vi "ConvertToArray.vi"(8 "error in (no error)":errorcluster, 11 "Cluster":T1) -> (0 "error out":errorcluster, 3 "Array":dbl[](array[numeric]))   [LabVIEW 2014]
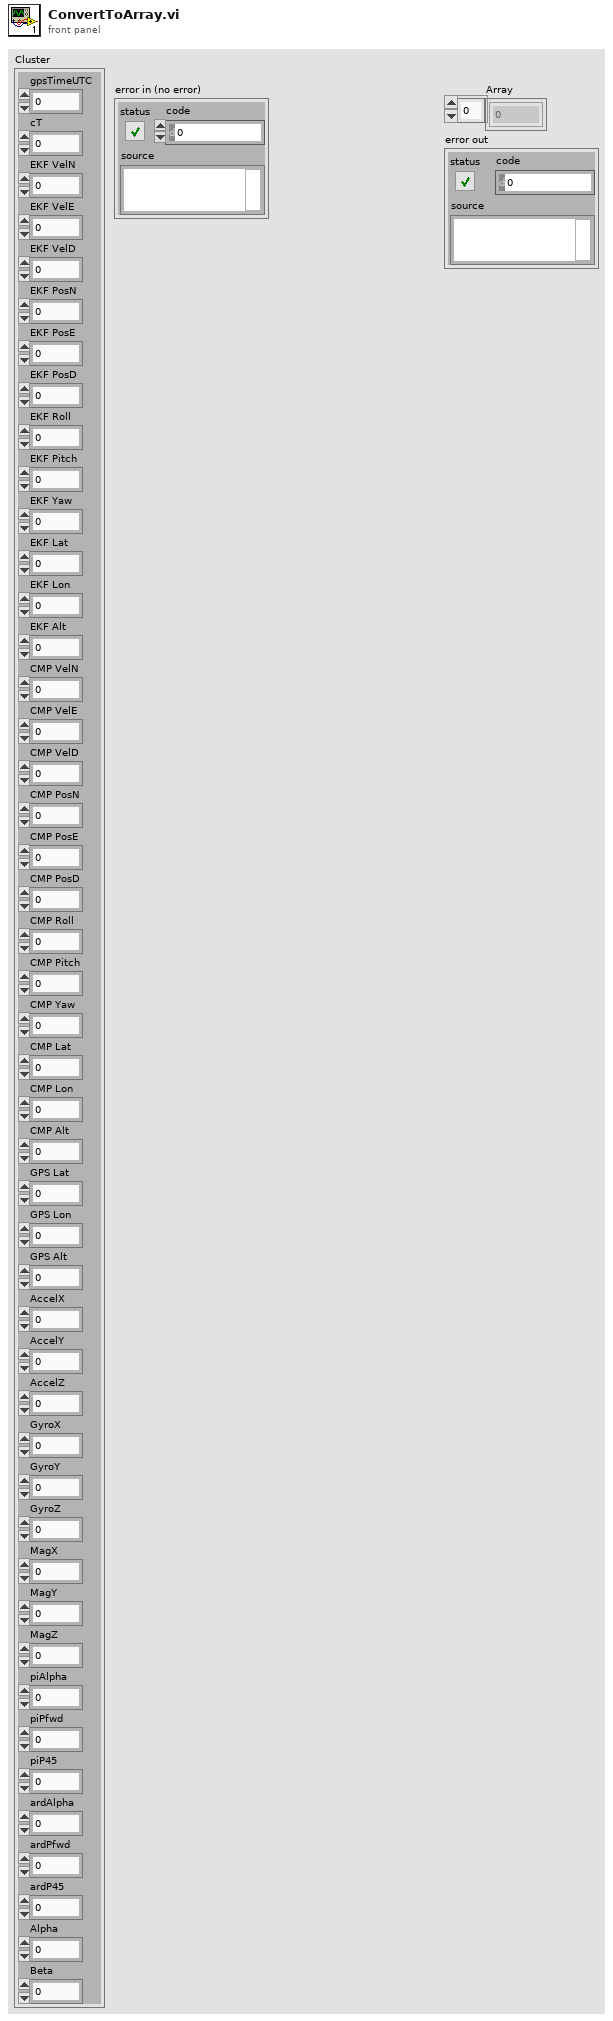
[diagram p1: front panel]
types:
  T1 = cluster{"gpsTimeUTC":i64, "cT":dbl, "EKF VelN":sgl, "EKF VelE":sgl, "EKF VelD":sgl, "EKF PosN":sgl, "EKF PosE":sgl, "EKF PosD":sgl, "EKF Roll":sgl, "EKF Pitch":sgl, "EKF Yaw":sgl, "EKF Lat":dbl, "EKF Lon":dbl, "EKF Alt":sgl, "CMP VelN":sgl, "CMP VelE":sgl, "CMP VelD":sgl, "CMP PosN":sgl, "CMP PosE":sgl, "CMP PosD":sgl, "CMP Roll":sgl, "CMP Pitch":sgl, "CMP Yaw":sgl, "CMP Lat":dbl, "CMP Lon":dbl, "CMP Alt":sgl, "GPS Lat":dbl, "GPS Lon":dbl, "GPS Alt":sgl, "AccelX":sgl, "AccelY":sgl, "AccelZ":sgl, "GyroX":sgl, "GyroY":sgl, "GyroZ":sgl, "MagX":sgl, "MagY":sgl, "MagZ":sgl, "piAlpha":sgl, "piPfwd":u16, "piP45":u16, "ardAlpha":sgl, "ardPfwd":u16, "ardP45":u16, "Alpha":sgl, "Beta":sgl}
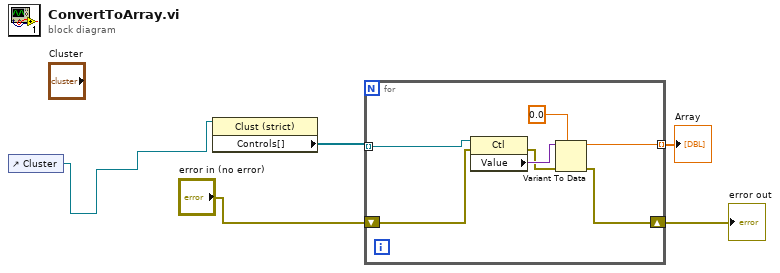
[diagram p0: block diagram]
diagram:
  n1 = control-ref of="Cluster"() -> (w1:refnum<vi>)
  n2 = property class="Clust (strict)"(reference=w1) -> ("Controls[]"=w2:refnum<vi>[])  [unwired: 1 in, 2 out]
  n3 = for {
    tunnel: w2 -> [w12] mode=indexing
    tunnel: [w9] -> w5 mode=indexing
    shift-right: [w6] -> w3
    shift-left: "error in (no error)" -> [w7]
    n4 = property class="Ctl"(reference=w12, error in=w7) -> (error out=w8:errorcluster, "Value"=w11:variant)  [unwired: 1 out]
    n5 = Variant To Data(error in=w8, type=0.0, Variant=w11) -> (data=w9:dbl, error out=w6:errorcluster)
  }
  "Array" <- w5
  "error out" <- w3
